vi "Call Chain to Key.vi"(8 "error in (no error)":errorcluster, 10 "Call Chain":string[](array[string]), 11 "Test Event Storage in":refnum<class "Test Event Storage.lvclass">) -> (0 "error out":errorcluster, 2 "Key":string, 3 "Test Event Storage out":refnum<class "Test Event Storage.lvclass">)   [LabVIEW 2009, in "Caraya.lvlib" / "Test Event Storage.lvclass"]
uses:
  Test Event Storage.lvclass
  Caraya.lvlib
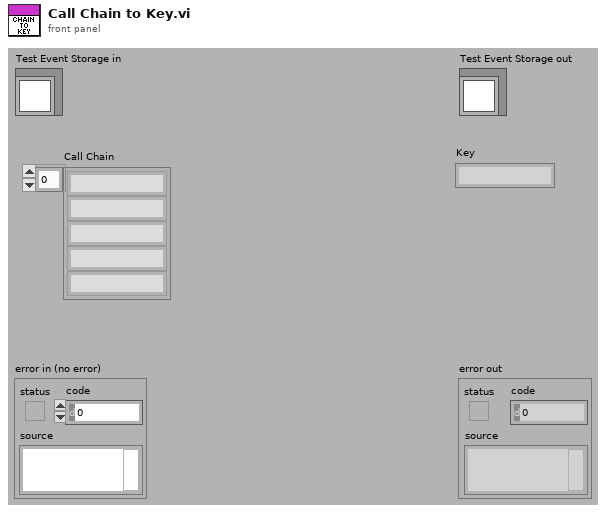
[diagram p1: front panel]
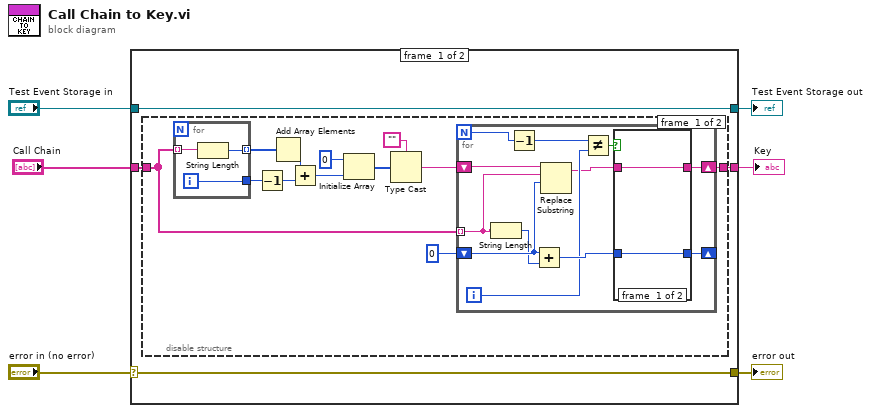
[diagram p0: block diagram]
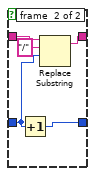
[diagram p2: hidden frame]
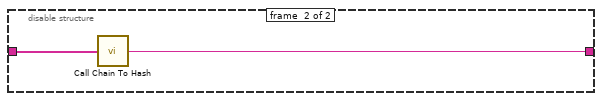
[diagram p3: hidden frame]
diagram:
  n1 = case shown="No Error" "error in (no error)" {
    selector: "error in (no error)" -> [w9 w48]
    tunnel: [w9 w48] -> w5
    tunnel: [w10 w47] -> w3
    tunnel: "Test Event Storage in" -> [w10 w47]
    tunnel: "Call Chain" -> [w8 _]
    tunnel: [w7 _] -> w1
    frame #0 {
      n2 = disable-structure shown="Enabled" {
        disable-tunnel: w8 -> [w14 w46]
        disable-tunnel: [w12 w45] -> w7
        frame #0 {
          n3 = for {
            tunnel: w14 -> [w44] mode=indexing
            tunnel: [w43] -> w20 mode=indexing
            tunnel: [w42] -> w22
            i -> [w42]
            n4 = String Length(string=w44) -> (length=w43:i32)
          }
          n5 = Decrement(x=w22) -> (x-1=w21:i32)
          n6 = Add Array Elements(numeric array=w20) -> (sum=w19:i32)
          n7 = Add(x=w19, y=w21) -> (x+y=w18:i32)
          n8 = Initialize Array(u8 0, w18) -> (w16:u8[])
          n9 = Type Cast(type="", x=w16) -> (*(type *) &x=w13:string)
          n10 = for {
            N -> [w31]
            tunnel: w14 -> [w32] mode=indexing
            shift-right: [w23] -> w12
            shift-left: w13 -> [w34]
            shift-right: [w27] -> _
            shift-left: 0 -> [w33]
            i -> [w26]
            n11 = String Length(string=w32) -> (length=w29:i32)
            n12 = Decrement(x=w31) -> (x-1=w30:i32)
            n13 = Add(x=w33, y=w29) -> (x+y=w28:i32)
            n14 = Replace Substring(3:w33, 4:w32, 5:w34) -> (1:w24:string)  [unwired: 1 in, 1 out]
            n15 = Not Equal?(x=w30, y=w26) -> (x != y?=w25:bool)
            n16 = case shown="True" w25 {
              tunnel: w28 -> [w36 w37]
              tunnel: [w36 w41] -> w27
              tunnel: w24 -> [w35 w40]
              tunnel: [w35 w39] -> w23
              frame #0 {
              }
              frame #1 {
                n17 = Increment(x=w37) -> (x+1=w41:i32)
                n18 = Replace Substring(3:w37, 4:"/" ("substring (\"\")"), 5:w40) -> (1:w39:string)  [unwired: 1 in, 1 out]
              }
            }
          }
        }
        frame #1 {
          n19 = call "Call Chain To Hash.vi"("VI Call Chain"=w46) -> ("Key"=w45:string)
        }
      }
    }
    frame #1 {
    }
  }
  "error out" <- w5
  "Test Event Storage out" <- w3
  "Key" <- w1
